vi "Enqueue Open Connection.vi"(8 "Error In":errorcluster, 11 "Name":string) -> (0 "Error Out":errorcluster, 2 "Connect?":bool)   [LabVIEW 2019, in "TCP2Foxconn.lvlib"]
uses:
  TCP2Foxconn.lvlib
  Queue/Queue.lvlib
  Data Error Notifier/Data and Error Notifier.lvlib
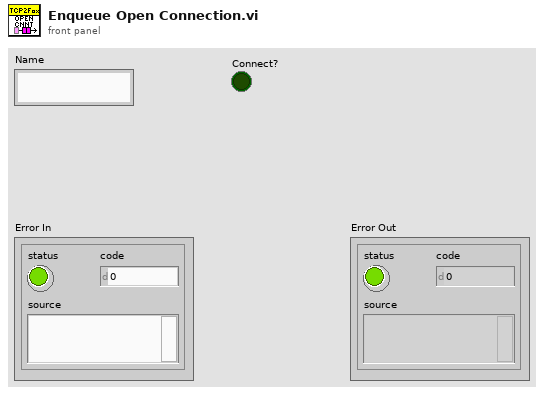
[diagram p1: front panel]
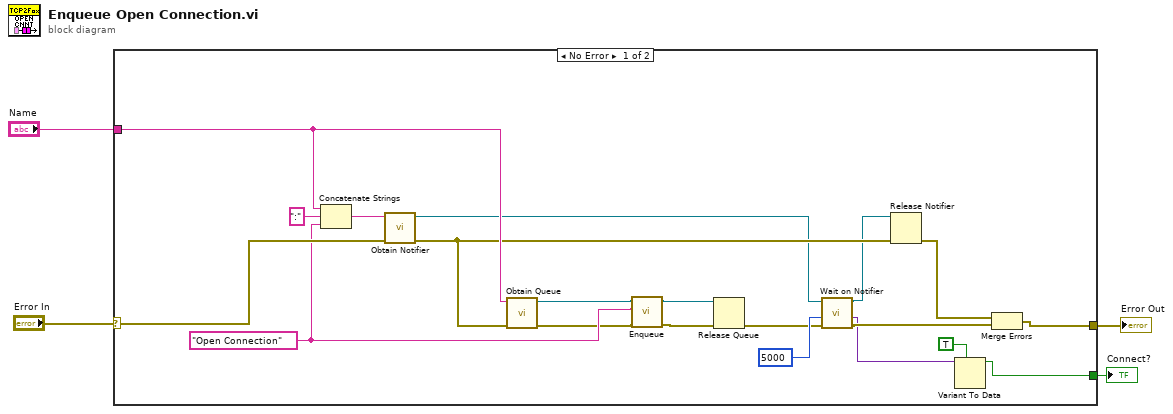
[diagram p0: block diagram]
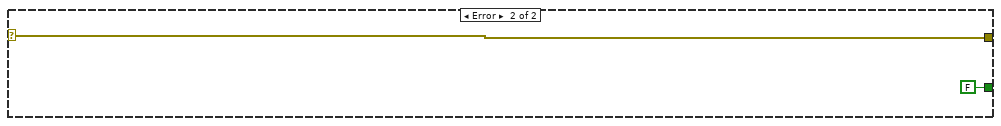
[diagram p2: hidden frame]
diagram:
  n1 = case shown="No Error" "Error In" {
    selector: "Error In" -> [w19 w26]
    tunnel: [w21 w26] -> w3
    tunnel: "Name" -> [w24 _]
    tunnel: [w5 FALSE] -> w1
    frame No Error {
      w16 = "Open Connection" ("Message")
      n2 = Concatenate Strings(w24, ":" ("string"), w16) -> (w20:string)
      n3 = call "Obtain Notifier.vi"("Error In"=w19, "Name"=w20) -> ("Error Out"=w18:errorcluster, "notifier out"=w12:refnum<notifier>)  [unwired: 8 in]
      n4 = call "Obtain Queue.vi"("Error In"=w18, "Name"=w24) -> ("Error Out"=w15:errorcluster, "queue out"=w17:refnum<queue>)  [unwired: 8 in]
      n5 = call "Enqueue.vi"("Error In"=w15, "Message"=w16, "queue in"=w17) -> ("Error Out"=w13:errorcluster, "queue out"=w14:refnum<queue>)  [unwired: 7 in]
      n6 = Release Queue(queue=w14, error in (no error)=w13) -> (error out=w10:errorcluster)  [unwired: 1 in, 2 out]
      n7 = call "Wait on Notifier.vi"("Error In"=w10, "timeout in ms (-1)"=5000, "notifier in"=w12) -> ("Error Out"=w8:errorcluster, "Data"=w7:variant, "notifier out"=w9:refnum<notifier>)  [unwired: 6 in]
      n8 = Release Notifier(notifier=w9, error in (no error)=w18) -> (error out=w22:errorcluster)  [unwired: 1 in, 2 out]
      n9 = Variant To Data(type=TRUE, Variant=w7) -> (data=w5:bool)  [unwired: 1 in, 1 out]
      n10 = Merge Errors(w22, w8) -> (w21:errorcluster)
    }
    frame Error {
    }
  }
  "Error Out" <- w3
  "Connect?" <- w1
